vi "ATF-Error Code source splitter.vi"(8 "error in (no error)":errorcluster) -> (2 "String":string, 3 "String 2":string)   [LabVIEW 2022 SP3]
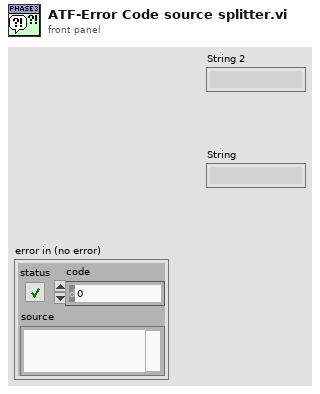
[diagram p1: front panel]
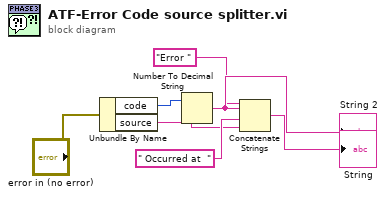
[diagram p0: block diagram]
diagram:
  n1 = Unbundle By Name("error in (no error)") -> ("code"=w2:i32, "source"=w1:string)
  n2 = Number To Decimal String(number=w2) -> (decimal integer string=w6:string)  [unwired: 1 out]
  "String 2" <- w6
  n3 = Concatenate Strings("Error " ("string"), w6, " Occurred at  " ("string"), w1) -> (→"String":string)
